vi "Assert Admin Controller.vi"() -> ()   [LabVIEW 2015, in "Admin_Actor.lvlib" / "Admin_Actor.lvclass"]
uses:
  Admin_Actor.lvclass
  API/_Database/Database.lvclass
  <vilib>/ActorFramework/Actor/Actor.lvclass
panel:
  in  "path":path=path "E:/哈工大竞技机器人队/机器人队管理系统/Database/CRTDatabase.accdb"
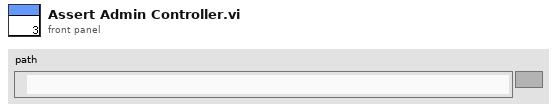
[diagram p1: front panel]
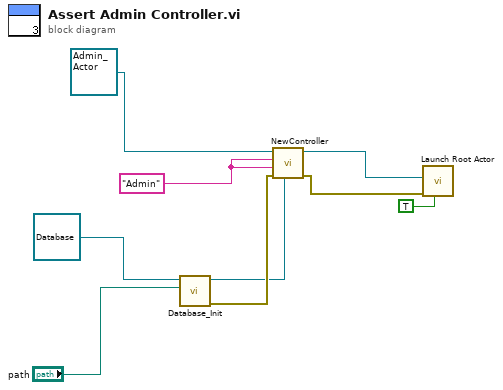
[diagram p0: block diagram]
diagram:
  w5 = "Admin" ("Name('')")
  n1 = call "Database_Init.vi"("path"="path", "object in"=refnum<class "Database.lvclass"> refnum ("Database")) -> ("error out"=w4:errorcluster, "object out"=w3:refnum<class "Database.lvclass">)  [unwired: 8 in]
  n2 = call-dynamic "NewController.vi"("Database"=w3, "error in (no error)"=w4, "Name('')"=w5, "ID(\"\")"=w5, "Admin_Actor in"=refnum<class "Admin_Actor.lvclass"> refnum) -> ("error out"=w2:errorcluster, "Admin_Actor out"=w1:refnum<class "Admin_Actor.lvclass">)  [unwired: 5 in]
  n3 = call <vilib>:"Launch Root Actor.vi"("Open Actor Core front panel? (F)"=TRUE, "error in (no error)"=w2, "Actor"=w1) -> ()  [unwired: 7 in, 2 out]
